vi "CRYLoad All Step Editor.vi"() -> ()   [LabVIEW 2013]
panel:
  in  "Pre Load":bool
  # "Load All Step Editor for speed."
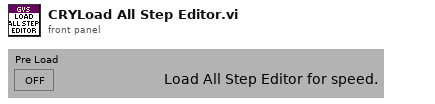
[diagram p1: front panel]
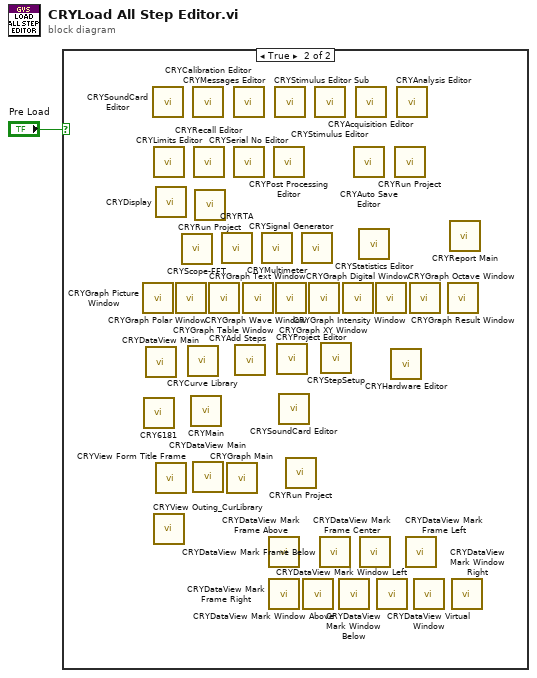
[diagram p0: block diagram]
diagram:
  n1 = case shown="True" "Pre Load" {
    frame False {
    }
    frame True {
      n2 = call "CRYGraph Picture Window.vi"() -> ()  [unwired: 12 in]
      n3 = call "CRY6181.vi"() -> ()  [unwired: 4 in]
      n4 = call "CRYDataView Main.vi"() -> ()  [unwired: 12 in]
      n5 = call "CRYSoundCard Editor.vi"() -> ()  [unwired: 12 in]
      n6 = call "CRYLimits Editor.vi"() -> ()  [unwired: 11 in, 1 out]
      n7 = call "CRYView Outing_CurLibrary.vi"() -> ()  [unwired: 12 in]
      n8 = call "CRYDisplay.vi"() -> ()  [unwired: 11 in, 5 out]
      n9 = call "CRYView Form Title Frame.vi"() -> ()  [unwired: 12 in]
      n10 = call "CRYGraph Polar Window.vi"() -> ()  [unwired: 12 in]
      n11 = call "CRYScope-FFT.vi"() -> ()  [unwired: 15 in, 5 out]
      n12 = call "CRYCurve Library.vi"() -> ()  [unwired: 12 in]
      n13 = call "CRYMain.vi"() -> ()  [unwired: 1 in]
      n14 = call "CRYCalibration Editor.vi"() -> ()  [unwired: 12 in]
      n15 = call "CRYDataView Main.vi"() -> ()  [unwired: 12 in]
      n16 = call "CRYRecall Editor.vi"() -> ()  [unwired: 12 in]
      n17 = call "CRYRun Project.vi"() -> ()  [unwired: 16 in]
      n18 = call "CRYGraph Table Window.vi"() -> ()  [unwired: 12 in]
      n19 = call "CRYRTA.vi"() -> ()  [unwired: 10 in, 6 out]
      n20 = call "CRYGraph Main.vi"() -> ()  [unwired: 12 in]
      n21 = call "CRYMessages Editor.vi"() -> ()  [unwired: 12 in]
      n22 = call "CRYSerial No Editor.vi"() -> ()  [unwired: 12 in]
      n23 = call "CRYAdd Steps.vi"() -> ()  [unwired: 12 in]
      n24 = call "CRYGraph Text Window.vi"() -> ()  [unwired: 12 in]
      n25 = call "CRYMultimeter.vi"() -> ()  [unwired: 12 in, 8 out]
      n26 = call "CRYDataView Mark Frame Above.vi"() -> ()  [unwired: 1 in]
      n27 = call "CRYDataView Mark Frame Right.vi"() -> ()  [unwired: 1 in]
      n28 = call "CRYPost Processing Editor.vi"() -> ()  [unwired: 12 in]
      n29 = call "CRYStimulus Editor Sub.vi"() -> ()  [unwired: 7 in, 3 out]
      n30 = call "CRYGraph Wave Window.vi"() -> ()  [unwired: 12 in]
      n31 = call "CRYProject Editor.vi"() -> ()  [unwired: 1 in]
      n32 = call "CRYSoundCard Editor.vi"() -> ()  [unwired: 12 in]
      n33 = call "CRYRun Project.vi"() -> ()  [unwired: 16 in]
      n34 = call "CRYSignal Generator.vi"() -> ()  [unwired: 11 in, 5 out]
      n35 = call "CRYDataView Mark Window Above.vi"() -> ()  [unwired: 1 in]
      n36 = call "CRYGraph XY Window.vi"() -> ()  [unwired: 12 in]
      n37 = call "CRYStimulus Editor.vi"() -> ()  [unwired: 12 in]
      n38 = call "CRYDataView Mark Frame Below.vi"() -> ()  [unwired: 1 in]
      n39 = call "CRYStepSetup.vi"() -> ()  [unwired: 1 in]
      n40 = call "CRYDataView Mark Window Below.vi"() -> ()  [unwired: 1 in]
      n41 = call "CRYGraph Digital Window.vi"() -> ()  [unwired: 12 in]
      n42 = call "CRYAuto Save Editor.vi"() -> ()  [unwired: 12 in]
      n43 = call "CRYAcquisition Editor.vi"() -> ()  [unwired: 12 in]
      n44 = call "CRYStatistics Editor.vi"() -> ()  [unwired: 12 in]
      n45 = call "CRYDataView Mark Frame Center.vi"() -> ()  [unwired: 1 in]
      n46 = call "CRYGraph Intensity Window.vi"() -> ()  [unwired: 12 in]
      n47 = call "CRYDataView Mark Window Left.vi"() -> ()  [unwired: 1 in]
      n48 = call "CRYHardware Editor.vi"() -> ()  [unwired: 12 in]
      n49 = call "CRYRun Project.vi"() -> ()  [unwired: 16 in]
      n50 = call "CRYAnalysis Editor.vi"() -> ()  [unwired: 12 in]
      n51 = call "CRYDataView Mark Frame Left.vi"() -> ()  [unwired: 1 in]
      n52 = call "CRYGraph Octave Window.vi"() -> ()  [unwired: 12 in]
      n53 = call "CRYDataView Virtual Window.vi"() -> ()  [unwired: 1 in]
      n54 = call "CRYGraph Result Window.vi"() -> ()  [unwired: 12 in]
      n55 = call "CRYReport Main.vi"() -> ()  [unwired: 2 in]
      n56 = call "CRYDataView Mark Window Right.vi"() -> ()  [unwired: 1 in]
    }
  }
